vi "Run VI.vi"(8 "Error In":errorcluster, 11 "Model In":refnum<class "Model.lvclass">) -> (0 "Error Out":errorcluster, 3 "Model out":refnum<class "Model.lvclass">)   [LabVIEW 2021, in "Model.lvclass"]
doc: "This VI runs the Analog To Digital Convertor VI ."
uses:
  Model.lvclass
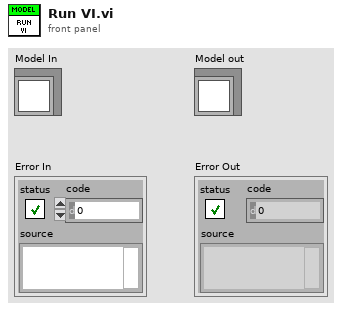
[diagram p1: front panel]
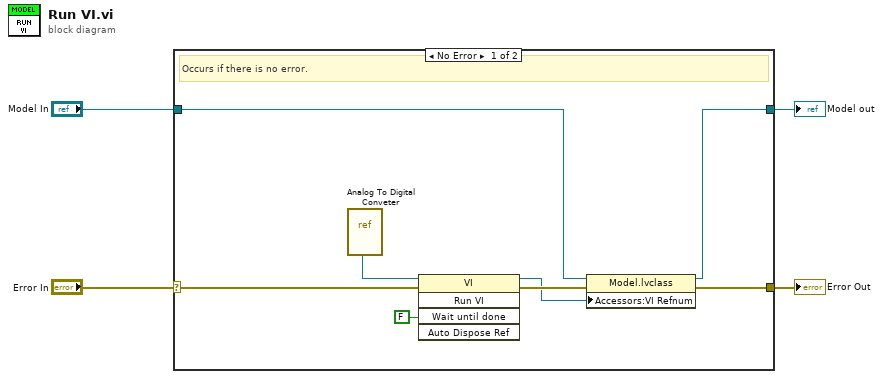
[diagram p0: block diagram]
diagram:
  n1 = case shown="No Error" "Error In" {
    selector: "Error In" -> [w10 w14]
    tunnel: [w8 w14] -> w3
    tunnel: [w6 w13] -> w1
    tunnel: "Model In" -> [w7 w13]
    frame No Error {
      # "Occurs if there is no error."
      n2 = vi-ref "Analog To Digital Conveter.vi"() -> (w12:refnum<vi>)
      n3 = invoke class="VI" method="Run VI"(reference=w12, error in=w10, "Wait until done"=FALSE ("Wait Until Done")) -> (reference out=w5:refnum<vi>, error out=w9:errorcluster)  [unwired: 2 in, 3 out]
      n4 = property class="Model.lvclass"(reference=w7, error in=w9, "Accessors:VI Refnum"=w5) -> (reference out=w6:refnum<class "Model.lvclass">, error out=w8:errorcluster)
    }
    frame Error {
      # "Occurs if there is any error."
    }
  }
  "Error Out" <- w3
  "Model out" <- w1
